vi "Read Gains.vi"(8 "error in (no error)":errorcluster, 11 "RTL-SDR in":refnum<class "Session.lvclass">) -> (0 "error out":errorcluster, 3 "RTL-SDR out":refnum<class "Session.lvclass">)   [LabVIEW 2020, in "RTL-SDR.lvlib" / "Session.lvclass"]
uses:
  Session.lvclass
  Session.lvclass/Session.ctl
  lib/librtlsdr.dll
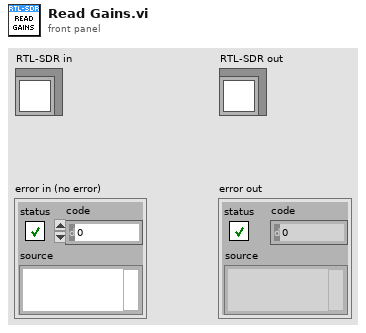
[diagram p1: front panel]
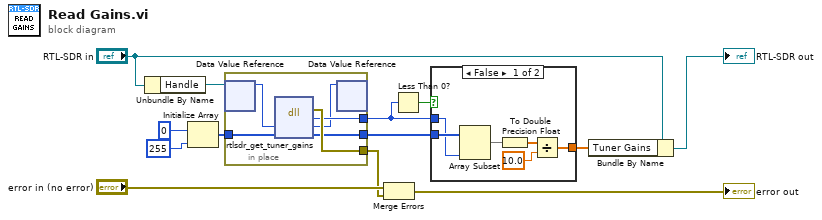
[diagram p0: block diagram]
diagram:
  n1 = Unbundle By Name("RTL-SDR in") -> ("Handle"=w1:refnum<data-value>)
  n2 = Initialize Array(0 ("element"), 255 ("dimension size")) -> (w4:i32[])
  n3 = in-place {
    in-place-border: [w18] -> w10
    in-place-border: w4 -> [w17]
    in-place-border: [w16] -> w3
    in-place-border: [w19] -> w2
    n4 = in-place-dvr #1(w1) -> (w15:u64)  [unwired: 1 out]
    n5 = dll-call lib="C:/dev/IlluminatedG/lv-rtl-sdr/lib/librtlsdr.dll" fn="rtlsdr_get_tuner_gains"("dev"=w15, "gains"=w17) -> (error out=w19:errorcluster, "return type"=w18:i32, "dev"=w14:u64, "gains"=w16:i32[])  [unwired: 3 in, 1 out]
    n6 = in-place-dvr #1(w14) -> ()  [unwired: 2 out]
  }
  n7 = Merge Errors("error in (no error)", w2) -> (→"error out":errorcluster)
  n8 = Less Than 0?(x=w10) -> (x < 0?=w11:bool)
  n9 = case shown="False" w11 {
    tunnel: w10 -> [w21 _]
    tunnel: [w23 _] -> w8
    tunnel: w3 -> [w22 _]
    frame False {
      n10 = Array Subset(array=w22, length=w21) -> (w20:i32[])  [unwired: 1 in]
      n11 = To Double Precision Float(number=w20) -> (double precision float=w25:dbl[])
      n12 = Divide(x=w25, y=10.0) -> (x/y=w23:dbl[])
    }
    frame True {
    }
  }
  n13 = Bundle By Name(cluster="RTL-SDR in", "Tuner Gains"=w8) -> (→"RTL-SDR out":refnum<class "Session.lvclass">)
